vi "FW LoadMMB0.vi"(8 "error in (no error)":errorcluster, 10 "Boot file":path, 11 "VISA resource name":refnum<visa-resource-name>) -> (0 "error out":errorcluster)   [LabVIEW 2010, in "lib1299.lvlib"]
uses:
  lib1299.lvlib
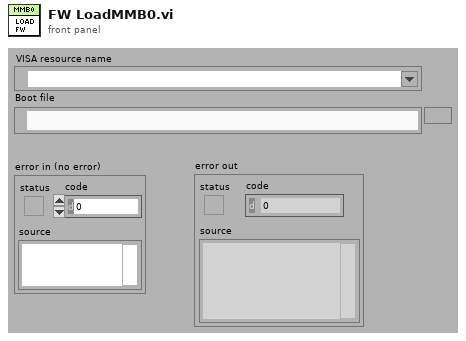
[diagram p1: front panel]
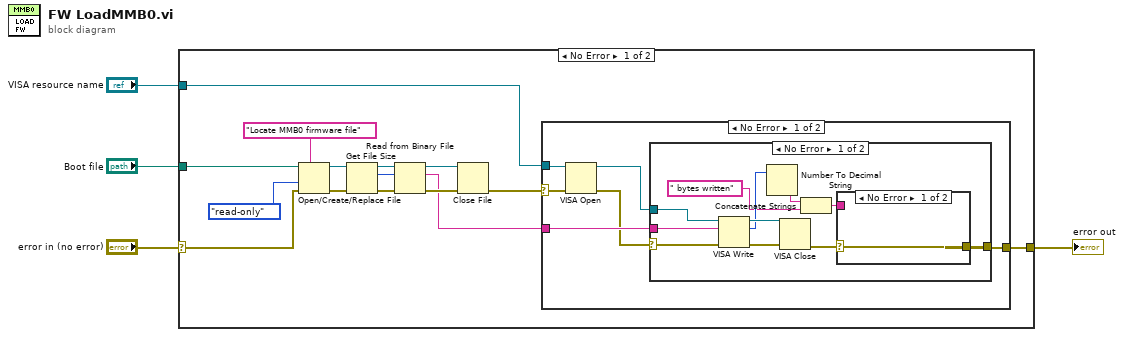
[diagram p0: block diagram]
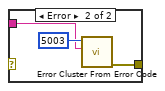
[diagram p2: hidden frame]
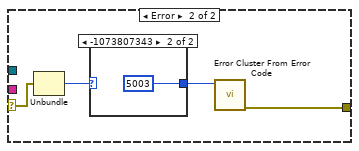
[diagram p3: hidden frame]
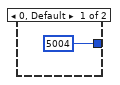
[diagram p4: hidden frame]
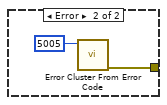
[diagram p5: hidden frame]
diagram:
  n1 = case shown="No Error" "error in (no error)" {
    selector: "error in (no error)" -> [w5 w49]
    tunnel: [w15 w49] -> w4
    tunnel: "Boot file" -> [w7 _]
    tunnel: "VISA resource name" -> [w6 _]
    frame No Error {
      n2 = Open/Create/Replace File(file path (use dialog)=w7, error in=w5, prompt="Locate MMB0 firmware file", access (0:read/write)=enum16{"read/write", "read-only", "write-only"}."read-only") -> (refnum out=w11:refnum<file>, error out=w13:errorcluster)  [unwired: 2 in, 1 out]
      n3 = Get File Size(file=w11, error in=w13) -> (refnum out=w10:refnum<file>, size (in bytes)=w9:i64, 0:w12:errorcluster)
      n4 = Read from Binary File(8:w12, 10:w9, 11:w10) -> (0:w18:errorcluster, 2:w16:string, 3:w19:refnum<file>)  [unwired: 3 in, 1 out]
      n5 = Close File(refnum=w19, error in=w18) -> (error out=w17:errorcluster)  [unwired: 1 out]
      n6 = case shown="No Error" w17 {
        selector: w17 -> [w24 _]
        tunnel: [w23 w47] -> w15
        tunnel: w6 -> [w25 _]
        tunnel: w16 -> [w21 _]
        frame No Error {
          n7 = VISA Open(error in (no error)=w24, VISA resource name=w25) -> (VISA resource name=w22:refnum<visa-resource-name>, error out=w20:errorcluster)  [unwired: 3 in]
          n8 = case shown="No Error" w20 {
            selector: w20 -> [w30 w43]
            tunnel: [w34 w44] -> w23
            tunnel: w22 -> [w33 _]
            tunnel: w21 -> [w31 _]
            frame No Error {
              n9 = VISA Write(VISA resource name=w33, write buffer=w31, error in (no error)=w30) -> (VISA resource name out=w32:refnum<visa-resource-name>, return count=w29:u32, error out=w36:errorcluster)
              n10 = Number To Decimal String(number=w29) -> (decimal integer string=w28:string)  [unwired: 1 in]
              n11 = VISA Close(VISA resource name=w32, error in (no error)=w36) -> (error out=w35:errorcluster)
              n12 = Concatenate Strings(w28, " bytes written" ("string")) -> (w26:string)
              n13 = case shown="No Error" w35 {
                selector: w35 -> [w37 _]
                tunnel: [w37 w39] -> w34
                tunnel: w26 -> [_ w38]
                frame No Error {
                }
                frame Error {
                  n14 = call <vilib>:"Error Cluster From Error Code.vi"("error message (\"\")"=w38, "error code (0)"=5003) -> ("error out"=w39:errorcluster)  [unwired: 7 in]
                }
              }
            }
            frame Error {
              n15 = Unbundle(w43) -> ("code"=w42:i32)  [unwired: 2 out]
              n16 = case shown="-1073807343" w42 {
                tunnel: [5004 ("error code (0)") 5003 ("error code (0)")] -> w41
                frame 0, Default {
                }
                frame -1073807343 {
                }
              }
              n17 = call <vilib>:"Error Cluster From Error Code.vi"("error code (0)"=w41) -> ("error out"=w44:errorcluster)  [unwired: 8 in]
            }
          }
        }
        frame Error {
          n18 = call <vilib>:"Error Cluster From Error Code.vi"("error code (0)"=5005) -> ("error out"=w47:errorcluster)  [unwired: 8 in]
        }
      }
    }
    frame Error {
    }
  }
  "error out" <- w4
